vi "Global SCELTA LINEA.vi"() -> ()   [LabVIEW 2019]
panel:
  in  "LINEA":T1(ring)
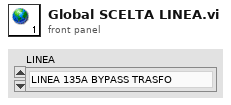
[diagram p1: front panel]
types:
  T1 = enum16{"LINEA 135A BYPASS TRASFO", "LINEA 15A BYPASS TRASFO", "LINEA 135A TRASFO 400V", "LINEA 135A TRASFO 500V", "LINEA 15A TRASFO 400V", "LINEA 15A TRASFO 500V", "LINEA 2", "NESSUNA LINEA SELEZIONATA"}
diagram:
